vi "Set SigGen State.vi"(8 "error in (no error)":errorcluster, 10 "Enable RF Output":bool, 11 "VISA Refnum in":refnum<visa-resource-name>) -> (0 "error out":errorcluster, 3 "VISA Refnum out":refnum<visa-resource-name>)   [LabVIEW 2015]
uses:
  <instrlib>/Agilent PSG MXG Series/Agilent PSG MXG Series.lvlib
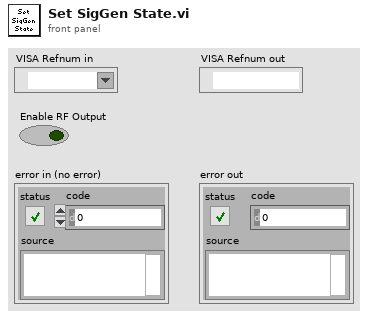
[diagram p1: front panel]
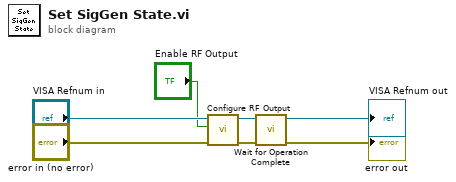
[diagram p0: block diagram]
diagram:
  n1 = call <instrlib>:"Configure RF Output.vi"("error in (no error)"="error in (no error)", "Enable RF Output (F:Disable)"="Enable RF Output", "VISA resource name"="VISA Refnum in") -> ("error out"=w6:errorcluster, "VISA resource name out"=w7:refnum<visa-resource-name>)  [unwired: 5 in, 2 out]
  n2 = call <instrlib>:"Wait for Operation Complete.vi"("error in (no error)"=w6, "VISA resource name"=w7) -> ("error out"=→"error out":errorcluster, "VISA resource name out"=→"VISA Refnum out":refnum<visa-resource-name>)  [unwired: 8 in]
